vi "Config Zero Mode.vi"(8 "error in":errorcluster, 10 "Zero Mode (off)":bool, 11 "VISA resource name":refnum<visa-resource-name>) -> (0 "error out":errorcluster, 3 "VISA resource name out":refnum<visa-resource-name>)   [LabVIEW 2016, in "Andeen-Hagerling 2550.lvlib"]
doc: "This VI changes the result mode between Absolute result mode and Zero compensation result mode."
uses:
  Andeen-Hagerling 2550.lvlib
panel:
  # "Zero Mode Properties"
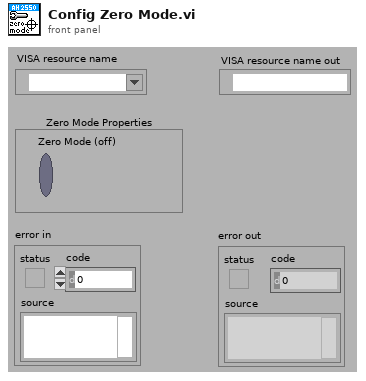
[diagram p1: front panel]
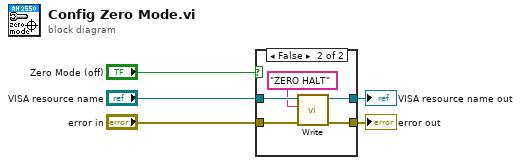
[diagram p0: block diagram]
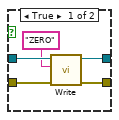
[diagram p2: hidden frame]
diagram:
  n1 = case shown="False" "Zero Mode (off)" {
    tunnel: "VISA resource name" -> [w10 w15]
    tunnel: "error in" -> [w9 w14]
    tunnel: [w8 w13] -> w3
    tunnel: [w7 w12] -> w2
    frame True {
      n2 = call "Write.vi"("error in"=w9, "command"="ZERO", "VISA resource name"=w10) -> ("error out"=w7:errorcluster, "VISA resource name out"=w8:refnum<visa-resource-name>)  [unwired: 7 in]
    }
    frame False {
      n3 = call "Write.vi"("error in"=w14, "command"="ZERO HALT", "VISA resource name"=w15) -> ("error out"=w12:errorcluster, "VISA resource name out"=w13:refnum<visa-resource-name>)  [unwired: 7 in]
    }
  }
  "VISA resource name out" <- w3
  "error out" <- w2
